vi "Plot Helper (Matrix).vi"(4 "Plot ID":i32, 6 "z matrix":sgl[][](array[numeric]), 8 "error in (no error)":errorcluster, 9 "y vector":sgl[](array[numeric]), 10 "x vector":sgl[](array[numeric]), 11 "3D Plot lvclass Array in":refnum<class "3D Plot Datatype.lvclass">[](array[class])) -> (0 "error out":errorcluster, 3 "3D Plot lvclass Array out":refnum<class "3D Plot Datatype.lvclass">[](array[class]))   [LabVIEW 2020, in "3D Comet Datatype.lvclass"]
doc: "Creates an animated graph with a circle that follows the data points. Multiple references to this VI generate multiple plots for the same graph."
uses:
  <vilib>/Math Plots/3D Math Plots/3D Comet/3D Comet Datatype/3D Comet Datatype.lvclass
  <vilib>/Math Plots/3D Math Plots/3D Plot/3D Plot Datatype/3D Plot Datatype.lvclass
  e:/builds/penguin/labview/branches/2020/dev/dist/vi.lib/Math Plots/3D Math Plots/3D Plot/3D Plot Datatype/3D Plot Datatype.lvclass
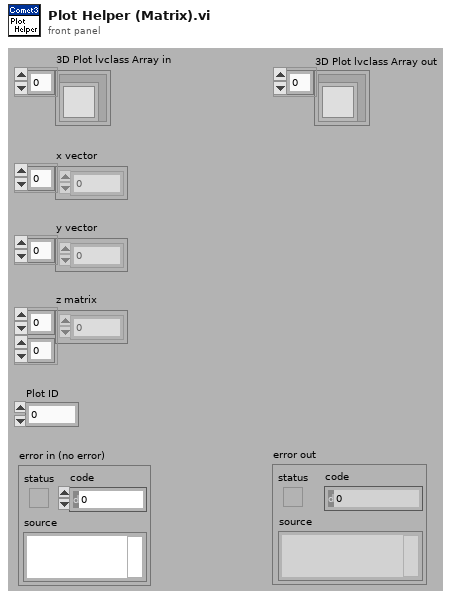
[diagram p1: front panel]
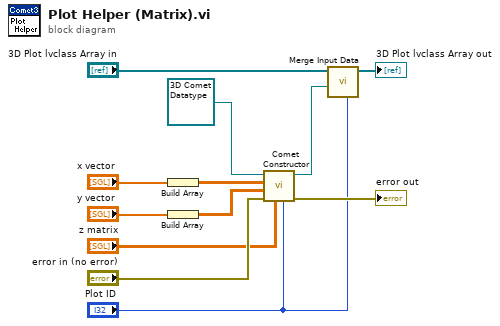
[diagram p0: block diagram]
diagram:
  n1 = Build Array("x vector") -> (w2:sgl[][])
  n2 = Build Array("y vector") -> (w1:sgl[][])
  n3 = call <vilib>:"Comet Constructor.vi"("Plot ID"="Plot ID", "z matrix"="z matrix", "error in (no error)"="error in (no error)", "y matrix"=w1, "x matrix"=w2, "3D Comet Datatype.lvclass in"=refnum<class "3D Comet Datatype.lvclass"> refnum ("3D Stem Datatype.lvclass")) -> ("error out"=→"error out":errorcluster, "3D Comet Datatype.lvclass out"=w7:refnum<class "3D Comet Datatype.lvclass">)  [unwired: 4 out]
  n4 = call <vilib>:"Merge Input Data.vi"("Plot ID"="Plot ID", "3D Plot lvclass in"=w7, "3D Plot lvclass Array in"="3D Plot lvclass Array in") -> ("3D Plot lvclass Array out"=→"3D Plot lvclass Array out":refnum<class "3D Plot Datatype.lvclass">[])  [unwired: 8 out]
